vi "CONEX-ALL Get Controller's address v2.vi"(11 "Connection Cluster in":T1) -> (1 "Controller's address":string, 3 "Connection Cluster out":T1)   [LabVIEW 2013]
doc: "SA? - Get controller's RS-485 address\n\nQuery current address of controller.\n\nReturn: Address of controller."
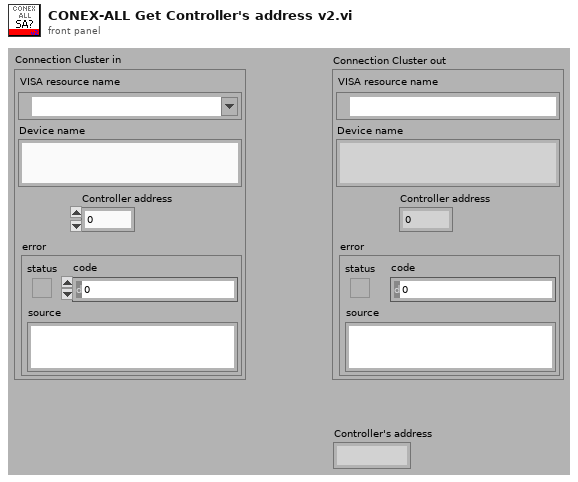
[diagram p1: front panel]
types:
  T1 = cluster{"VISA resource name":refnum<visa-resource-name>, "Device name":string, "Controller address":i32, "error":errorcluster}
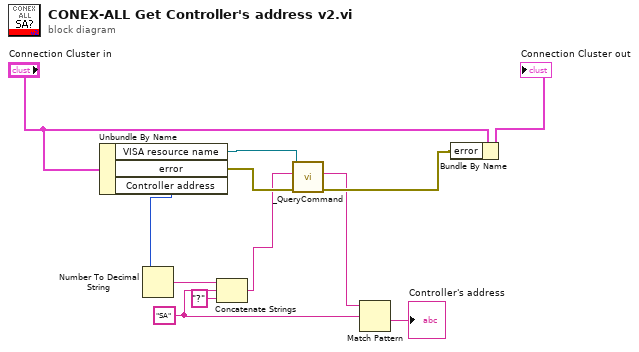
[diagram p0: block diagram]
diagram:
  w10 = "SA" ("strCommand")
  n1 = Unbundle By Name("Connection Cluster in") -> ("VISA resource name"=w8:refnum<visa-resource-name>, "error"=w6:errorcluster, "Controller address"=w1:i32)
  n2 = Number To Decimal String(number=w1) -> (decimal integer string=w12:string)  [unwired: 1 out]
  n3 = Concatenate Strings(w12, w10, "?" ("chaîne")) -> (w3:string)
  n4 = call "_QueryCommand.vi"("error in"=w6, "Command"=w3, "Instrument Channel in"=w8) -> ("error out"=w7:errorcluster, "Response"=w2:string)  [unwired: 6 in, 1 out]
  n5 = Match Pattern(string=w2, regular expression=w10) -> (after substring=→"Controller's address":string)  [unwired: 4 out]
  n6 = Bundle By Name(cluster="Connection Cluster in", "error"=w7) -> (→"Connection Cluster out":T1)
